vi "Approximate Polygon (Convex Hull).vi"(5 "Ensure Convex? (Default: True)":bool=TRUE, 7 "Epsilon % (Default: -1 Do Not Use)":dbl=-1.0 format="%#_13g", 8 "error in (no error)":errorcluster, 10 "Number of Sides":u8, 11 "Points in":T1[](array[typedef])) -> (0 "error out":errorcluster, 3 "Points out":T1[](array[typedef]))   [LabVIEW 2020, in "shape.lvlib"]
uses:
  shape.lvlib
  common/Image Point (Integer).ctl
  common/common.lvlib
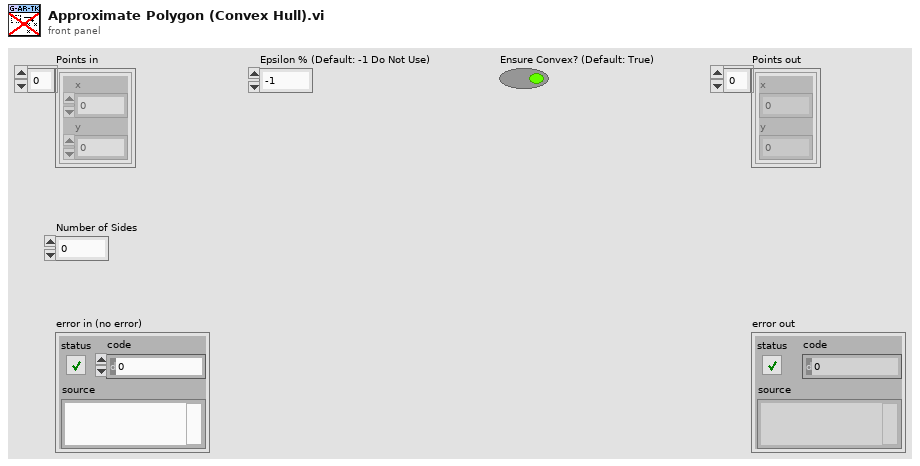
[diagram p1: front panel]
types:
  T1 = typedef "common.lvlib/Image Point (Integer).ctl" = cluster{"x":i32, "y":i32}
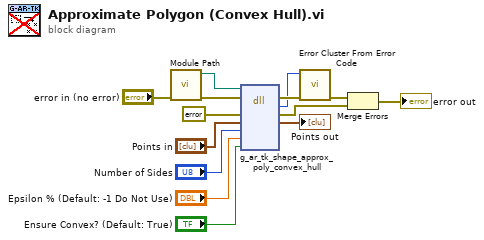
[diagram p0: block diagram]
diagram:
  n1 = call "Module Path.vi"("error in (no error)"="error in (no error)") -> ("error out"=w3:errorcluster, "Path"=w2:path)  [unwired: 9 in]
  n2 = dll-call lib="?" fn="g_ar_tk_shape_approx_poly_convex_hull" ("g_ar_toolkit.*.*:g_ar_tk_image_draw_line")(path in=w2, error in=w3, "error_cluster"=errorcluster {"status"=FALSE, "code"=0, "source"=""} ("error constant"), "points"="Points in", "n_sides"="Number of Sides", "epsilon_pct"="Epsilon % (Default: -1 Do Not Use)", "ensure_convex"="Ensure Convex? (Default: True)") -> (error out=w12:errorcluster, "MgErr"=w11:i32, "error_cluster"=w8:errorcluster, "points"=→"Points out":T1[])  [unwired: 4 in, 1 out]
  n3 = call <vilib>:"Error Cluster From Error Code.vi"("error in (no error)"=w12, "error code (0)"=w11) -> ("error out"=w10:errorcluster)  [unwired: 7 in]
  n4 = Merge Errors(w10, w8) -> (→"error out":errorcluster)
